vi "Tag Metadata Organize Tags.vi"(0 "Current Tags":string[][](array[string]), 11 "Group Index":i32) -> (8 "Display Tags":string[][](array[string]))   [LabVIEW 2020]
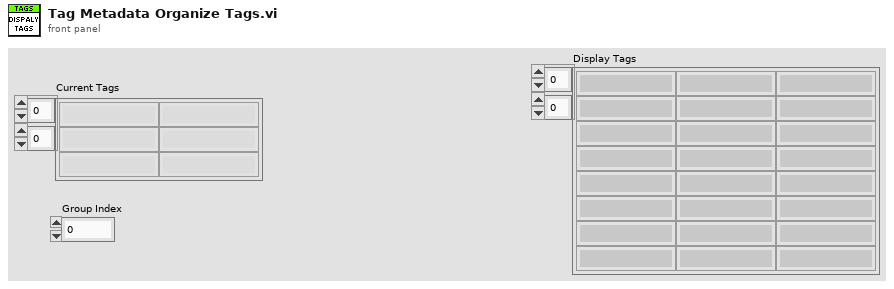
[diagram p1: front panel]
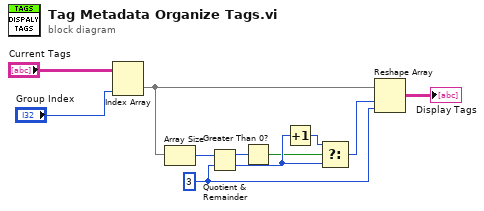
[diagram p0: block diagram]
diagram:
  w5 = 3 ("y")
  n1 = Index Array(array="Current Tags", index (col)="Group Index") -> (element=w4:string[])  [unwired: 1 in]
  n2 = Array Size(array=w4) -> (size(s)=w6:i32)
  n3 = Quotient & Remainder(x=w6, y=w5) -> (x-y*floor(x/y)=w7:i32, floor(x/y)=w9:i32)
  n4 = Greater Than 0?(x=w7) -> (x > 0?=w8:bool)
  n5 = Increment(x=w9) -> (x+1=w10:i32)
  n6 = Select(t=w10, s=w8, f=w9) -> (s? t:f=w11:i32)
  n7 = Reshape Array(w4, w11, w5) -> (→"Display Tags":string[][])
